vi "Velmex.Vi"(1 "Command String":string="F,C,I1M1000", 3 "Motor":u8=1, 4 "Distance":i16=100) -> ()   [LabVIEW 2014]
doc: "This is a \"quick-run\" node to help use the Velmex 2-axis stepper motor controllers.\n\nThe Serial Port number for the USB emulator seems to always be \"5\".\n\nYou can choose to either type in an entire command string, or to specify a particular motor and direction.\nThe command string is formatted as \"F,C,I1M1000\" (for example), as specified in the Velmex documentation. You can send multiple commands in this mode.\n\nOr, you can simply specify a single motor (1 or 2) with an amount of travel (such as 200, or -300, etc.)."
panel:
  in  "Port":i32=1 min=1 max=255 step=1
  out "PortStatus":bool
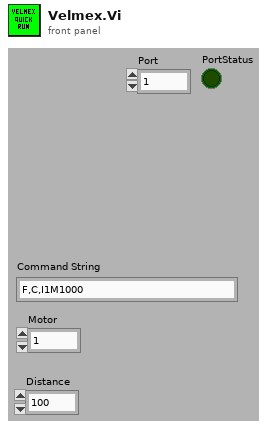
[diagram p1: front panel]
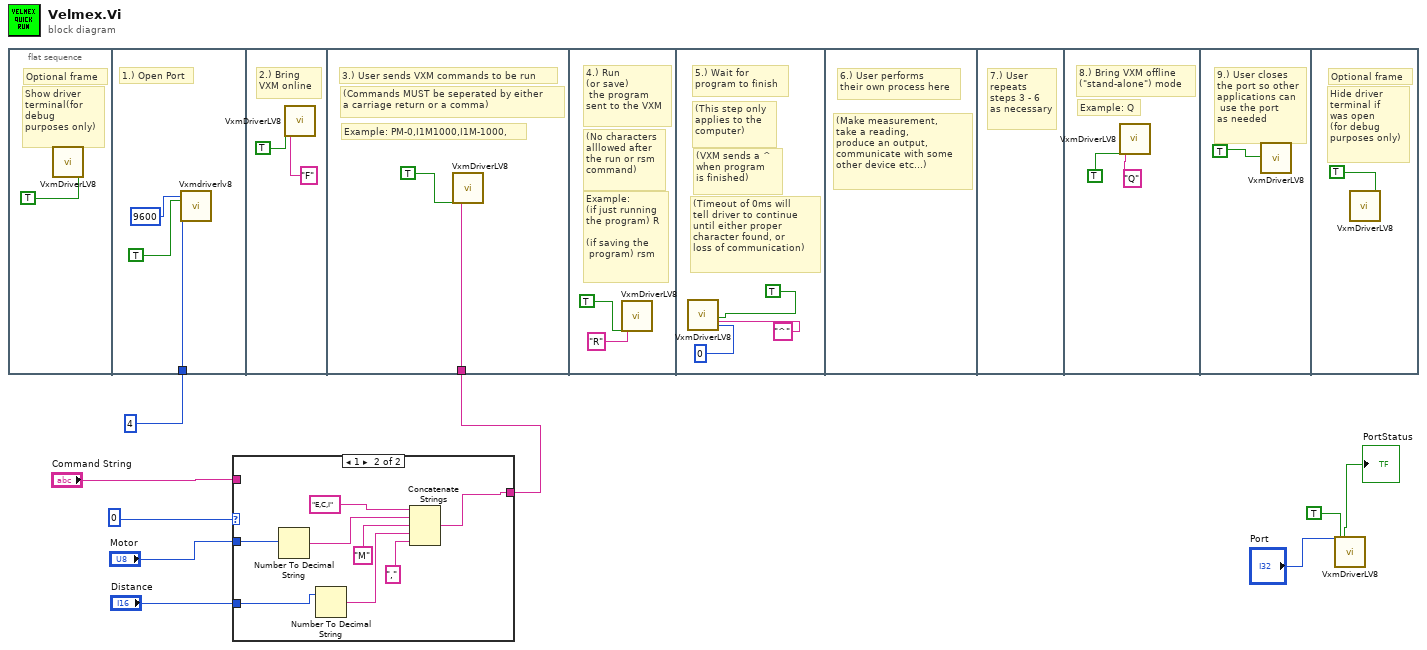
[diagram p0: block diagram]
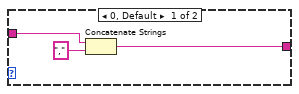
[diagram p2: hidden frame]
diagram:
  n1 = flat-sequence {
    tunnel: u8 4 ("Serial Port #") -> [w11]
    tunnel: w8 -> [w16]
    frame #0 {
      # "Show driver\nterminal(for\ndebug \npurposes only)"
      # "Optional frame"
      n2 = call "VxmDriverLV8.vi"("Show Terminal"=TRUE) -> ()  [unwired: 21 in, 6 out]
    }
    frame #1 {
      # "1.) Open Port"
      n3 = call "Vxmdriverlv8.Vi"("Port"=w11, "Baud Rate"=9600, "Open Port"=TRUE) -> ()  [unwired: 19 in, 6 out]
    }
    frame #2 {
      # "2.) Bring\nVXM online"
      n4 = call "VxmDriverLV8.vi"("Send\nchars\nto port"=TRUE, "Chars to send"="F") -> ()  [unwired: 20 in, 6 out]
    }
    frame #3 {
      # "(Commands MUST be seperated by either\na carriage return or a comma)"
      # "Example: PM-0,I1M1000,I1M-1000,"
      # "3.) User sends VXM commands to be run"
      n5 = call "VxmDriverLV8.vi"("Send\nchars\nto port"=TRUE, "Chars to send"=w16) -> ()  [unwired: 20 in, 6 out]
    }
    frame #4 {
      # "Example:\n(if just running \nthe program) R\n\n(if saving the\n program) rsm"
      # "(No characters\nalllowed after \nthe run or rsm \ncommand)"
      # "4.) Run \n(or save)\n the program \nsent to the VXM"
      n6 = call "VxmDriverLV8.vi"("Send\nchars\nto port"=TRUE, "Chars to send"="R") -> ()  [unwired: 20 in, 6 out]
    }
    frame #5 {
      # "(Timeout of 0ms will\ntell driver to continue\nuntil either proper \ncharacter found, or\nloss of communication)"
      # "(VXM sends a ^ \nwhen program \nis finished)"
      # "(This step only \napplies to the \ncomputer)"
      # "5.) Wait for \nprogram to finish"
      n7 = call "VxmDriverLV8.vi"("Wait\nfor \nchar"=TRUE, "Char(s) to wait for"="^", "Char\nTimeout\nTime (ms)"=0) -> ()  [unwired: 19 in, 6 out]
    }
    frame #6 {
      # "(Make measurement,\ntake a reading,\nproduce an output, \ncommunicate with some \nother device etc...)"
      # "6.) User performs \ntheir own process here"
    }
    frame #7 {
      # "7.) User\nrepeats \nsteps 3 - 6\nas necessary"
    }
    frame #8 {
      # "Example: Q"
      # "8.) Bring VXM offline \n(\"stand-alone\") mode"
      n8 = call "VxmDriverLV8.vi"("Send\nchars\nto port"=TRUE, "Chars to send"="Q") -> ()  [unwired: 20 in, 6 out]
    }
    frame #9 {
      # "9.) User closes\nthe port so other\napplications can\n use the port\nas needed"
      n9 = call "VxmDriverLV8.vi"("Close Port"=TRUE) -> ()  [unwired: 21 in, 6 out]
    }
    frame #10 {
      # "Hide driver\nterminal if\nwas open\n(for debug \npurposes only)"
      # "Optional frame"
      n10 = call "VxmDriverLV8.vi"("Hide Terminal"=TRUE) -> ()  [unwired: 21 in, 6 out]
    }
  }
  n11 = case shown="1" u16 0 ("Command Mode") {
    tunnel: [w27 w37] -> w8
    tunnel: "Command String" -> [w28 _]
    tunnel: "Motor" -> [_ w35]
    tunnel: "Distance" -> [_ w33]
    frame 0, Default {
      n12 = Concatenate Strings(w28, "," ("string")) -> (w27:string)
    }
    frame 1 {
      n13 = Number To Decimal String(number=w35) -> (decimal integer string=w34:string)  [unwired: 1 in]
      n14 = Number To Decimal String(number=w33) -> (decimal integer string=w32:string)  [unwired: 1 in]
      n15 = Concatenate Strings("E,C,I", w34, "M", w32, ",") -> (w37:string)
    }
  }
  n16 = call "VxmDriverLV8.vi"("Port"="Port", "Is Port Open"=TRUE) -> ("Port\nOpen\nStatus"=→"PortStatus":bool)  [unwired: 20 in, 5 out]
